vi "tap_stim_rec_async.vi"(0 "Convert Power to Voltage B":bool, 2 "voltages/power B":dbl[](array[numeric]), 3 "SSH password":string, 4 "Transfer and Run Date Folder After Experiment":bool, 5 "SSH user name":string, 6 "Tags":string, 7 "Frames":i32, 8 "Convert Power to Voltage A":bool, 9 "voltages/power A":dbl[](array[numeric]), 10 "parameters":string[](array[string]), 11 "parameters headers":string[](array[string])) -> ()   [LabVIEW 2019]
uses:
  <vilib>/Utility/file.llb/Write To Spreadsheet File (string).vi
  <vilib>/Utility/file.llb/Read From Spreadsheet File (string).vi
  <vilib>/vision/driver/IMAQdx.llb/IMAQdx Acquisition Mode.ctl
  <vilib>/vision/driver/NI_Vision_Acquisition_Software.lvlib
  <vilib>/userdefined/High Color/IMAQdx.ctl
  <vilib>/vision/driver/IMAQdx.llb/IMAQdx Buffer Number Mode.ctl
  <vilib>/Utility/file.llb/Write To Spreadsheet File (DBL).vi
panel:
  out "Saved Buffer Number":u32
  out "ProcessFrameRate":dbl
  out "# elements in queue":i32
  out "CameraFrameRate":dbl
  out "Camera Buffer Number":u32
  out "Image":T1(plugin-control)
  out "JPEG Quality":dbl
  out "Error":string
  out "Save Directory":path
  in  "stop":bool
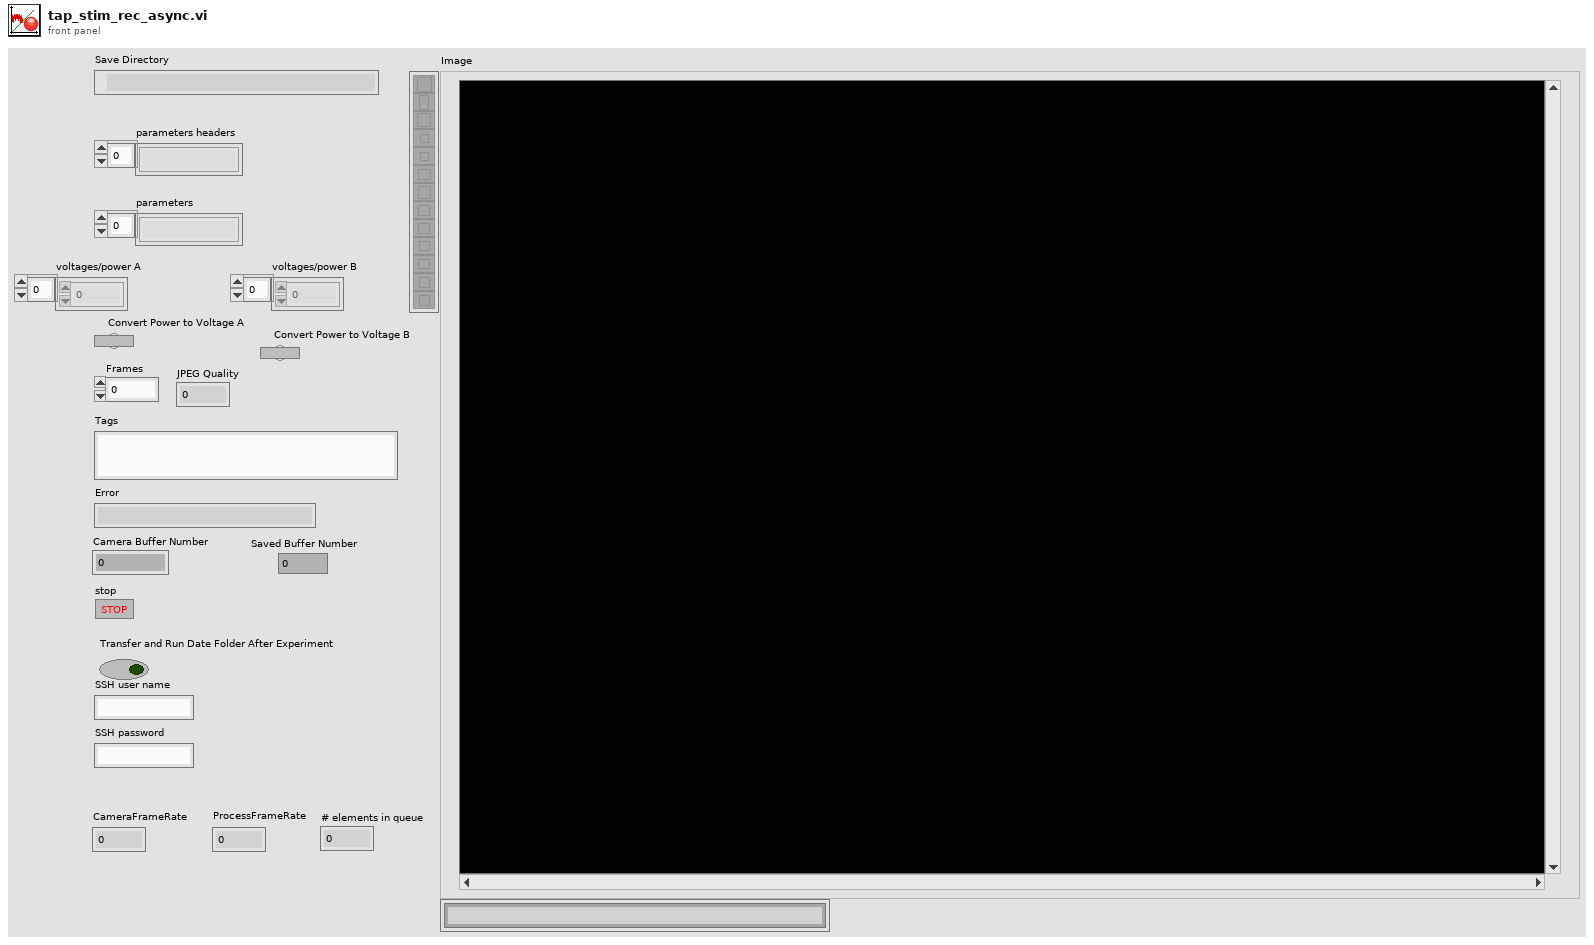
[diagram p1: front panel]
types:
  T1 = typedef "IMAQ Image.ctl" = refnum<image>
  T2 = typedef "IMAQdx.ctl" = refnum<k21>
  T3 = typedef "NI_Vision_Acquisition_Software.lvlib/IMAQdx Buffer Number Mode.ctl" = enum32{"Next", "Last", "Buffer Number", "Every", "Last New"}
  T4 = typedef "Image Type" = u32
  T5 = typedef "NI_Vision_Acquisition_Software.lvlib/IMAQdx Acquisition Mode.ctl" = enum32{"One Shot", "Continuous"}
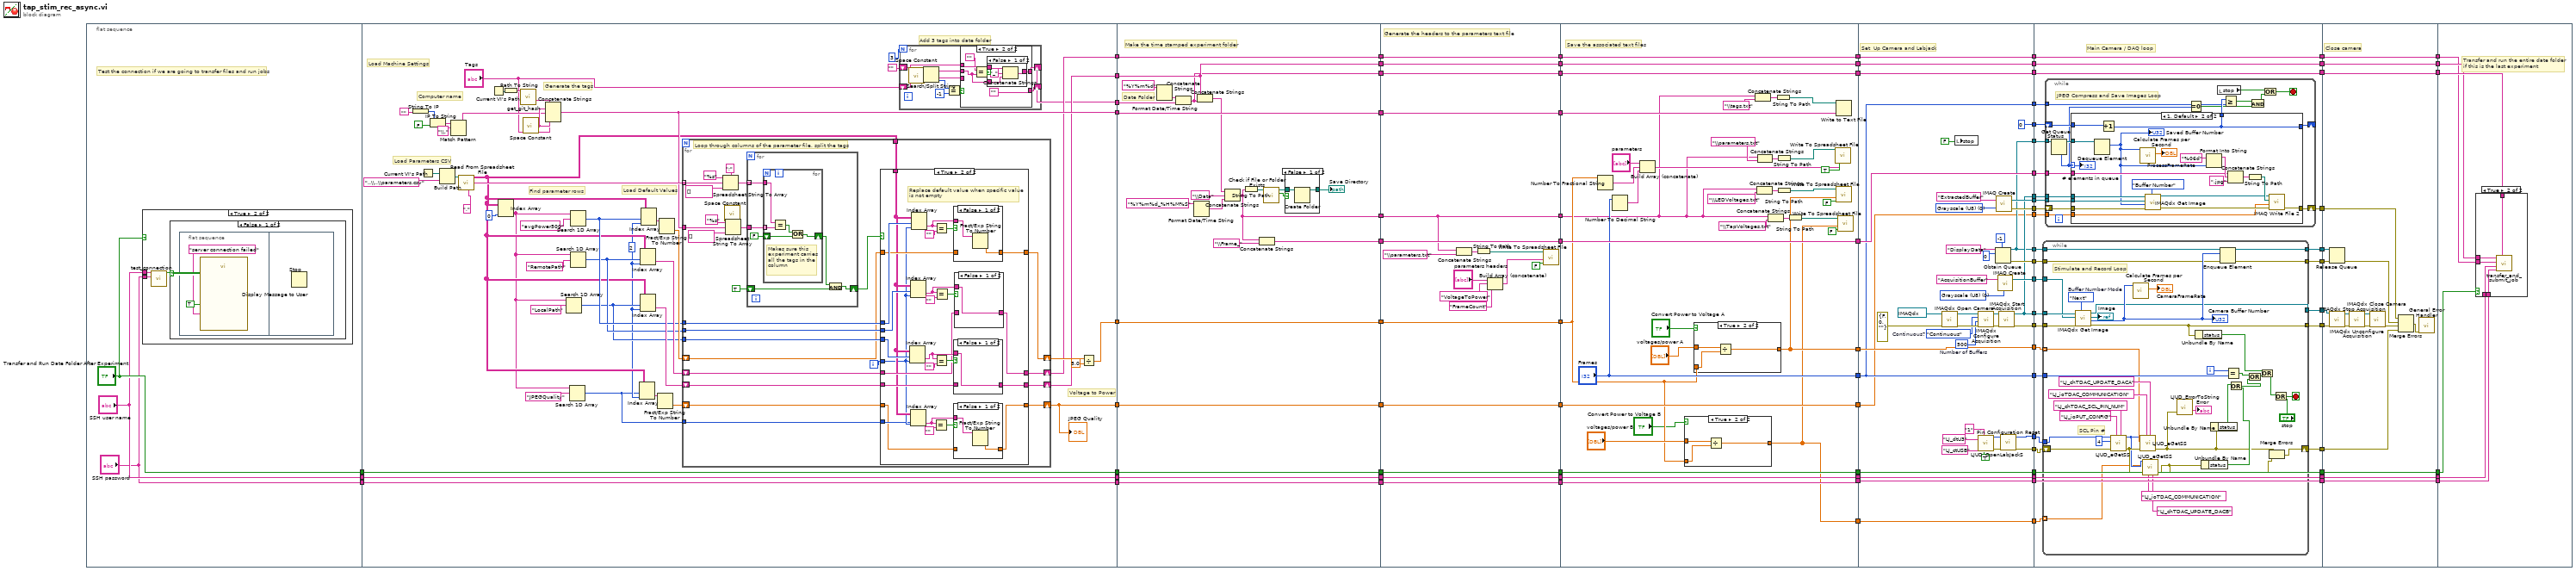
[diagram p0: block diagram]
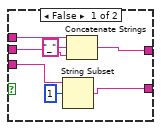
[diagram p4: hidden frame]
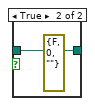
[diagram p11: hidden frame]
diagram:
  n1 = flat-sequence {
    tunnel: ["Transfer and Run Date Folder After Experiment"] -> w50
    tunnel: ["SSH user name"] -> w49
    tunnel: ["SSH password"] -> w48
    tunnel: [w134] -> w80
    tunnel: [w117] -> w79
    tunnel: [w108] -> w70
    tunnel: [w109] -> w69
    tunnel: w50 -> [w126]
    tunnel: w49 -> [w125]
    tunnel: w48 -> [w124]
    tunnel: [w126] -> w41
    tunnel: [w125] -> w34
    tunnel: [w124] -> w33
    tunnel: [w105] -> w26
    tunnel: [w96] -> w25
    tunnel: [w270] -> w64
    tunnel: [w269] -> w62
    tunnel: [w268] -> w60
    tunnel: [w267] -> w58
    tunnel: [w249] -> w56
    tunnel: [w251] -> w54
    tunnel: [w266] -> w52
    tunnel: w69 -> [w266]
    tunnel: w70 -> [w251]
    tunnel: w79 -> [w267]
    tunnel: w80 -> [w268]
    tunnel: [w258] -> w42
    tunnel: w41 -> [w258]
    tunnel: [w257] -> w35
    tunnel: w34 -> [w257]
    tunnel: w33 -> [w256]
    tunnel: [w256] -> w32
    tunnel: w26 -> [w252]
    tunnel: w25 -> [w248]
    tunnel: [w248] -> w22
    tunnel: w64 -> [w292]
    tunnel: [w292] -> w63
    tunnel: w62 -> [w278]
    tunnel: [w278] -> w61
    tunnel: w60 -> [w291]
    tunnel: [w291] -> w59
    tunnel: w58 -> [w290]
    tunnel: [w290] -> w57
    tunnel: w56 -> [w289]
    tunnel: [w289] -> w55
    tunnel: w54 -> [w288]
    tunnel: [w288] -> w53
    tunnel: w52 -> [w287]
    tunnel: [w287] -> w51
    tunnel: [w277] -> w43
    tunnel: w42 -> [w277]
    tunnel: [w276] -> w36
    tunnel: w35 -> [w276]
    tunnel: w32 -> [w275]
    tunnel: [w275] -> w31
    tunnel: [w274] -> w23
    tunnel: w22 -> [w274]
    tunnel: w63 -> [w327]
    tunnel: [w327] -> w85
    tunnel: [w298] -> w83
    tunnel: ["Frames"] -> w82
    tunnel: w61 -> [w294]
    tunnel: w59 -> [w301]
    tunnel: w57 -> [w305]
    tunnel: w55 -> [w316]
    tunnel: [w316] -> w75
    tunnel: [w315] -> w71
    tunnel: w53 -> [w315]
    tunnel: [w314] -> w65
    tunnel: w51 -> [w314]
    tunnel: [w308] -> w44
    tunnel: w43 -> [w308]
    tunnel: [w307] -> w37
    tunnel: w36 -> [w307]
    tunnel: w31 -> [w306]
    tunnel: [w306] -> w30
    tunnel: [w304] -> w24
    tunnel: w23 -> [w304]
    tunnel: [w293] -> w1
    tunnel: w85 -> [w344]
    tunnel: [w374] -> w87
    tunnel: [w373] -> w86
    tunnel: [w377] -> w84
    tunnel: w83 -> [w377]
    tunnel: w82 -> [w343]
    tunnel: [w343] -> w81
    tunnel: [w371] -> w76
    tunnel: w75 -> [w371]
    tunnel: [w370] -> w72
    tunnel: w71 -> [w370]
    tunnel: [w369] -> w66
    tunnel: w65 -> [w369]
    tunnel: [w368] -> w45
    tunnel: w44 -> [w368]
    tunnel: [w367] -> w38
    tunnel: w37 -> [w367]
    tunnel: w30 -> [w366]
    tunnel: [w366] -> w29
    tunnel: w24 -> [w341]
    tunnel: [w350] -> w21
    tunnel: [w345] -> w20
    tunnel: [w349] -> w19
    tunnel: [w348] -> w18
    tunnel: [w342] -> w17
    tunnel: [w347] -> w14
    tunnel: [w346] -> w13
    tunnel: [w345] -> w12
    tunnel: [w344] -> w11
    tunnel: [w343] -> w10
    tunnel: [w342] -> w9
    tunnel: [w341] -> w8
    tunnel: [0] -> w4
    tunnel: [w338] -> w2
    tunnel: w1 -> [w338]
    tunnel: w87 -> [w395]
    tunnel: w86 -> [w387]
    tunnel: w84 -> [w393]
    tunnel: w81 -> [w394]
    tunnel: [w410] -> w77
    tunnel: w76 -> [w410]
    tunnel: [w409] -> w73
    tunnel: w72 -> [w409]
    tunnel: [w408] -> w67
    tunnel: w66 -> [w408]
    tunnel: [w407] -> w46
    tunnel: w45 -> [w407]
    tunnel: [w406] -> w39
    tunnel: w38 -> [w406]
    tunnel: w29 -> [w405]
    tunnel: [w405] -> w28
    tunnel: w21 -> [w388]
    tunnel: w20 -> [w389]
    tunnel: w19 -> [w390]
    tunnel: w18 -> [w391]
    tunnel: w17 -> [w392]
    tunnel: [w383] -> w16
    tunnel: [w382] -> w15
    tunnel: w14 -> [w404]
    tunnel: w13 -> [w403]
    tunnel: w12 -> [w402]
    tunnel: w11 -> [w401]
    tunnel: w10 -> [w400]
    tunnel: w9 -> [w399]
    tunnel: w8 -> [w398]
    tunnel: [w381] -> w7
    tunnel: [w384] -> w6
    tunnel: [w397] -> w5
    tunnel: w4 -> [w396]
    tunnel: [w385] -> w3
    tunnel: w2 -> [w386]
    tunnel: [w509] -> w78
    tunnel: w77 -> [w509]
    tunnel: [w508] -> w74
    tunnel: w73 -> [w508]
    tunnel: [w507] -> w68
    tunnel: w67 -> [w507]
    tunnel: [w506] -> w47
    tunnel: w46 -> [w506]
    tunnel: [w505] -> w40
    tunnel: w39 -> [w505]
    tunnel: w28 -> [w504]
    tunnel: [w504] -> w27
    tunnel: w16 -> [w499]
    tunnel: w15 -> [w498]
    tunnel: w7 -> [w493]
    tunnel: w6 -> [w496]
    tunnel: w5 -> [w495]
    tunnel: w3 -> [w494]
    tunnel: w78 -> [w515]
    tunnel: w74 -> [w514]
    tunnel: w68 -> [w513]
    tunnel: w47 -> [w512]
    tunnel: w40 -> [w511]
    tunnel: w27 -> [w510]
    frame #0 {
      # "Test the connection if we are going to transfer files and run jobs"
      n2 = case shown="True" "Transfer and Run Date Folder After Experiment" {
        tunnel: "SSH password" -> [_ w93]
        tunnel: "SSH user name" -> [_ w91]
        frame False {
        }
        frame True {
          n3 = call "test_connection.vi"("Username"=w91, "Password"=w93) -> ("Connection Successful"=w92:bool)  [unwired: 7 in]
          n4 = case shown="False" w92 {
            frame False {
              n5 = flat-sequence {
                frame #0 {
                  n6 = call "Display Message to User"("Enable"=TRUE, "Message"="server connection failed") -> ()  [unwired: 8 in, 2 out]
                }
                frame #1 {
                  n7 = Stop() -> ()  [unwired: 1 in]
                }
              }
            }
            frame True {
            }
          }
        }
      }
    }
    frame #1 {
      w99 = 2
      # "Add 3 tags into date folder"
      # "Generate the tags"
      # "Find parameter rows"
      # "Load Default Values"
      # "Voltage to Power"
      # "Load Parameters CSV"
      # "Computer name"
      # "Load Machine Settings"
      n8 = String To IP(1:"") -> (0:w142:u32)
      n9 = Current VI's Path() -> (path=w137:path)
      n10 = IP To String(1:FALSE, 2:w142) -> (0:w139:string)
      n11 = Build Path(base path=w137, name or relative path="..\\..\\parameters.csv") -> (appended path=w128:path)
      n12 = Match Pattern(string=w139, regular expression="\\.") -> (before substring=w119:string)  [unwired: 1 in, 3 out]
      n13 = call-poly <vilib>:"Read From Spreadsheet File.vi"("delimiter (\\t)"=",", "file path (dialog if empty)"=w128) -> ("first row"=w118:string[], "all rows"=w101:string[][])  [unwired: 5 in, 3 out]
      n14 = Current VI's Path() -> (path=w121:path)
      n15 = Index Array(array=w101, index (col)=0) -> (element=w100:string[])  [unwired: 1 in]
      n16 = Path To String(path=w121) -> (string=w120:string)
      n17 = call "get_git_hash.vi"("VI folder"=w120) -> ("github hash"=w123:string)  [unwired: 10 in]
      n18 = call <vilib>:"Space Constant.vi"() -> ("String"=w122:string)
      n19 = Concatenate Strings(w123, w122, w119, w122, "Tags") -> (w117:string)
      n20 = Search 1D Array(1D array=w100, element="LocalPath") -> (index of element=w111:i32)  [unwired: 1 in]
      n21 = Search 1D Array(1D array=w100, element="JPEGQuality") -> (index of element=w97:i32)  [unwired: 1 in]
      n22 = Search 1D Array(1D array=w100, element="RemotePath") -> (index of element=w112:i32)  [unwired: 1 in]
      n23 = Search 1D Array(1D array=w100, element="avgPower500") -> (index of element=w113:i32)  [unwired: 1 in]
      n24 = Index Array(array=w101, index (row)=w97, index (col)=w99) -> (element=w102:string)
      n25 = Index Array(array=w101, index (row)=w112, index (col)=w99) -> (element=w115:string)
      n26 = Index Array(array=w101, index (row)=w111, index (col)=w99) -> (element=w114:string)
      n27 = Index Array(array=w101, index (row)=w113, index (col)=w99) -> (element=w130:string)
      n28 = Fract/Exp String To Number(string=w102) -> (number=w98:dbl)  [unwired: 3 in, 1 out]
      n29 = Fract/Exp String To Number(string=w130) -> (number=w116:dbl)  [unwired: 3 in, 1 out]
      n30 = for {
        tunnel: w118 -> [w196] mode=indexing
        tunnel: w117 -> [w188]
        tunnel: w113 -> [w183]
        tunnel: w112 -> [w182]
        tunnel: w111 -> [w181]
        tunnel: w101 -> [w186]
        shift-right: [w178] -> w110
        shift-left: w116 -> [w179]
        shift-right: [w175] -> w109
        shift-left: w115 -> [w176]
        shift-right: [w174] -> w108
        shift-left: w114 -> [w177]
        shift-right: [w171] -> w96
        shift-left: w98 -> [w173]
        tunnel: w97 -> [w172]
        i -> [w180]
        # "Loop through columns of the parameter file, split the tags"
        n31 = Spreadsheet String To Array(delimiter (Tab)=";", format string="%s", spreadsheet string=w196, array type (2D Dbl)=string[] []) -> (array=w192:string[])
        n32 = call <vilib>:"Space Constant.vi"() -> ("String"=w190:string)
        n33 = Spreadsheet String To Array(delimiter (Tab)=w190, format string="%s", spreadsheet string=w188, array type (2D Dbl)=string[] []) -> (array=w187:string[])
        n34 = for {
          tunnel: w192 -> [w242] mode=indexing
          tunnel: w187 -> [w241]
          shift-right: [w239] -> w184
          shift-left: TRUE -> [w237]
          n35 = for {
            tunnel: w242 -> [w247]
            tunnel: w241 -> [w246] mode=indexing
            shift-right: [w243] -> w238
            shift-left: FALSE -> [w244]
            # "Makes sure this\nexperiment carries\nall the tags in the\ncolumn"
            n36 = Equal?(x=w247, y=w246) -> (x = y?=w245:bool)
            n37 = Or(x=w245, y=w244) -> (x .or. y?=w243:bool)
          }
          n38 = And(x=w238, y=w237) -> (x .and. y?=w239:bool)
        }
        n39 = case shown="True" w184 {
          tunnel: w179 -> [w200 w221]
          tunnel: [w200 w220] -> w178
          tunnel: w183 -> [_ w226]
          tunnel: w182 -> [_ w225]
          tunnel: w181 -> [_ w224]
          tunnel: w180 -> [_ w203]
          tunnel: w186 -> [_ w204]
          tunnel: [w199 w210] -> w175
          tunnel: [w198 w212] -> w174
          tunnel: w177 -> [w198 w211]
          tunnel: w176 -> [w199 w209]
          tunnel: w173 -> [w197 w201]
          tunnel: w172 -> [_ w202]
          tunnel: [w197 w205] -> w171
          frame False {
          }
          frame True {
            # "Replace default value when specific value\nis not empty"
            n40 = Index Array(array=w204, index (row)=w224, index (col)=w203) -> (element=w213:string)
            n41 = Index Array(array=w204, index (row)=w225, index (col)=w203) -> (element=w216:string)
            n42 = Index Array(array=w204, index (row)=w202, index (col)=w203) -> (element=w206:string)
            n43 = Index Array(array=w204, index (row)=w226, index (col)=w203) -> (element=w219:string)
            n44 = Equal?(x=w206, y="") -> (x = y?=w207:bool)
            n45 = Equal?(x=w219, y="") -> (x = y?=w222:bool)
            n46 = Equal?(x=w213, y="") -> (x = y?=w214:bool)
            n47 = Equal?(x=w216, y="") -> (x = y?=w217:bool)
            n48 = case shown="False" w207 {
              tunnel: w201 -> [_ w229]
              tunnel: [w228 w229] -> w205
              tunnel: w206 -> [w227 _]
              frame False {
                n49 = Fract/Exp String To Number(string=w227) -> (number=w228:dbl)  [unwired: 3 in, 1 out]
              }
              frame True {
              }
            }
            n50 = case shown="False" w222 {
              tunnel: w221 -> [_ w236]
              tunnel: [w235 w236] -> w220
              tunnel: w219 -> [w234 _]
              frame False {
                n51 = Fract/Exp String To Number(string=w234) -> (number=w235:dbl)  [unwired: 3 in, 1 out]
              }
              frame True {
              }
            }
            n52 = case shown="False" w214 {
              tunnel: w213 -> [w230 _]
              tunnel: [w230 w231] -> w212
              tunnel: w211 -> [_ w231]
              frame False {
              }
              frame True {
              }
            }
            n53 = case shown="False" w217 {
              tunnel: w216 -> [w232 _]
              tunnel: [w232 w233] -> w210
              tunnel: w209 -> [_ w233]
              frame False {
              }
              frame True {
              }
            }
          }
        }
      }
      "JPEG Quality" <- w96
      n54 = for {
        N: 3 -> [_]
        shift-right: [w143] -> _
        shift-left: "Tags" -> [w152]
        shift-right: [w145] -> w105
        shift-left: "" -> [w150]
        n55 = call <vilib>:"Space Constant.vi"() -> ("String"=w151:string)
        n56 = Search/Split String(string=w152, search string/char (-)=w151) -> (substring before match=w149:string, match + rest of string=w148:string, offset of match=w147:i32)  [unwired: 1 in]
        n57 = Equal?(x=w147, y=-1) -> (x = y?=w144:bool)
        n58 = case shown="True" w144 {
          tunnel: w150 -> [w153 w163]
          tunnel: w149 -> [w154 w160]
          tunnel: w148 -> [w155 _]
          tunnel: [w157 ""] -> w143
          tunnel: [w156 w162] -> w145
          frame False {
            n59 = String Subset(string=w155, offset (0)=1) -> (substring=w157:string)  [unwired: 1 in]
            n60 = Concatenate Strings(w153, "_", w154) -> (w156:string)
          }
          frame True {
            n61 = Equal?(x="", y=w160) -> (x = y?=w164:bool)
            n62 = case shown="False" w164 {
              tunnel: w163 -> [w167 w170]
              tunnel: [w168 w170] -> w162
              tunnel: w160 -> [w166 _]
              frame False {
                n63 = Concatenate Strings(w167, "_", w166) -> (w168:string)
              }
              frame True {
              }
            }
          }
        }
      }
      n64 = Divide(x=w110, y=5.0) -> (x/y=w134:dbl)
    }
    frame #2 {
      # "Make the time stamped experiment folder"
      # "Date Folder"
      n65 = Format Date/Time String(time format string (%c)="%Y%m%d") -> (date/time string=w253:string)  [unwired: 2 in]
      n66 = Concatenate Strings(w253, w252) -> (w249:string)
      n67 = Format Date/Time String(time format string (%c)="%Y%m%d_%H%M%S") -> (date/time string=w255:string)  [unwired: 2 in]
      n68 = Concatenate Strings(w251, w249) -> (w250:string)
      n69 = Concatenate Strings(w250, "\\Data", w255) -> (w269:string)
      n70 = String To Path(string=w269) -> (path=w261:path)
      n71 = Concatenate Strings(w269, "\\Frame_") -> (w270:string)
      n72 = call <vilib>:"Check if File or Folder Exists.vi"("path"=w261) -> ("file or folder exists?"=w264:bool, "dup path"=w263:path)  [unwired: 8 in, 1 out]
      n73 = case shown="False" w264 {
        tunnel: [w271 w273] -> w260
        tunnel: w263 -> [w272 w273]
        frame False {
          n74 = Create Folder(path (use dialog)=w272) -> (created path=w271:path)  [unwired: 2 in, 2 out]
        }
        frame True {
          (unwired) errorcluster {"status"=FALSE, "code"=0, "source"=""} ("error out")
        }
      }
      "Save Directory" <- w260
    }
    frame #3 {
      # "Generate the headers to the parameters text file"
      n75 = Concatenate Strings(w278, "\\parameters.txt") -> (w286:string)
      n76 = String To Path(string=w286) -> (path=w285:path)
      n77 = Build Array (concatenate)("parameters headers", "VoltageToPower", "FrameCount") -> (w282:string[])
      n78 = call-poly <vilib>:"Write To Spreadsheet File.vi"("append to file? (new file:F)"=FALSE, "1D data"=w282, "file path (dialog if empty)"=w285) -> ()  [unwired: 5 in, 1 out]
    }
    frame #4 {
      # "Save the associated text files"
      n79 = Number To Fractional String(number=w301) -> (F-format string=w310:string)  [unwired: 3 in]
      n80 = Number To Decimal String(number="Frames") -> (decimal integer string=w311:string)  [unwired: 1 in]
      n81 = Build Array (concatenate)("parameters", w310, w311) -> (w320:string[])
      n82 = case shown="True" "Convert Power to Voltage B" {
        tunnel: "voltages/power B" -> [w330 w333]
        tunnel: [w330 w331] -> w293
        tunnel: w301 -> [_ w332]
        frame False {
        }
        frame True {
          n83 = Divide(x=w333, y=w332) -> (x/y=w331:dbl[])
        }
      }
      n84 = case shown="True" "Convert Power to Voltage A" {
        tunnel: "voltages/power A" -> [w334 w337]
        tunnel: [w334 w335] -> w298
        tunnel: w301 -> [_ w336]
        frame False {
        }
        frame True {
          n85 = Divide(x=w337, y=w336) -> (x/y=w335:dbl[])
        }
      }
      n86 = Concatenate Strings(w294, "\\tags.txt") -> (w318:string)
      n87 = Concatenate Strings(w294, "\\LEDVoltages.txt") -> (w329:string)
      n88 = Concatenate Strings(w294, "\\parameters.txt") -> (w324:string)
      n89 = Concatenate Strings(w294, "\\TapVoltages.txt") -> (w297:string)
      n90 = String To Path(string=w318) -> (path=w317:path)
      n91 = String To Path(string=w329) -> (path=w328:path)
      n92 = String To Path(string=w324) -> (path=w323:path)
      n93 = String To Path(string=w297) -> (path=w295:path)
      n94 = call-poly <vilib>:"Write To Spreadsheet File.vi"("append to file? (new file:F)"=TRUE, "1D data"=w320, "file path (dialog if empty)"=w323) -> ()  [unwired: 5 in, 1 out]
      n95 = call-poly <vilib>:"Write To Spreadsheet File.vi"("append to file? (new file:F)"=FALSE, "1D data"=w298, "file path (dialog if empty)"=w328) -> ()  [unwired: 5 in, 1 out]
      n96 = Write to Text File(file (use dialog)=w317, text=w305) -> ()  [unwired: 2 in, 3 out]
      n97 = call-poly <vilib>:"Write To Spreadsheet File.vi"("append to file? (new file:F)"=FALSE, "1D data"=w293, "file path (dialog if empty)"=w295) -> ()  [unwired: 5 in, 1 out]
    }
    frame #5 {
      w353 = T4 0 items=["Grayscale (U8)", "Grayscale (I16)", "Grayscale (SGL)", "Complex (CSG)", "RGB (U32)", "HSL (U32)", "RGB (U64)"] ("Image Type")
      w362 = T4 0 items=["Grayscale (U8)", "Grayscale (I16)", "Grayscale (SGL)", "Complex (CSG)", "RGB (U32)", "HSL (U32)", "RGB (U64)"] ("Image Type")
      w363 = u32 500  # Number of Buffers
      w359 = IMAQdx_Acquisition_Mode."Continuous"  # Continuous?
      # "Set  Up Camera and Labjack"
      n98 = call <vilib>:"IMAQdx Open Camera.vi"("error in"=errorcluster {"status"=FALSE, "code"=0, "source"=""}, "Session In"=T2 "cam0") -> ("error out"=w364:errorcluster, "Session Out"=w365:T2)  [unwired: 8 in]
      n99 = local write "stop"(FALSE) -> ()
      n100 = call "LJUD_OpenLabJackS.vi"("FirstFound"=TRUE, "Address"="1" ("DeviceType"), "ConnectionType"="LJ_ctUSB", "DeviceType"="LJ_dtU3") -> ("error out"=w372:errorcluster, "Handle"=w375:i32)  [unwired: 5 in, 1 out]
      n101 = call <vilib>:"IMAQdx Configure Acquisition.vi"("error in"=w364, "Number of Buffers"=w363, "Continuous?"=w359, "Session In"=w365) -> ("error out"=w360:errorcluster, "Session Out"=w358:T2)  [unwired: 6 in]
      n102 = Obtain Queue(max queue size (-1, unlimited)=-1, name (unnamed)="DisplayData", element data type=u32 0) -> (queue out=w342:refnum<queue>, error out=w348:errorcluster)  [unwired: 2 in, 1 out]
      n103 = call "IMAQ Create"("Image Name"="ExtractedBuffer", "Image Type"=w353) -> ("New Image"=w346:T1, "error out"=w347:errorcluster)  [unwired: 3 in]
      n104 = call "IMAQ Create"("Image Name"="AcquisitionBuffer", "Image Type"=w362) -> ("New Image"=w349:T1)  [unwired: 3 in, 1 out]
      n105 = call <vilib>:"IMAQdx Start Acquisition.vi"("error in"=w360, "Session In"=w358) -> ("error out"=w350:errorcluster, "Session Out"=w345:T2)  [unwired: 8 in]
      n106 = call "Pin Configuration Reset.vi"("error in"=w372, "Handle In"=w375) -> ("error out"=w373:errorcluster, "Handle Out"=w374:i32)  [unwired: 8 in]
    }
    frame #6 {
      # "Main Camera / DAQ loop"
      n107 = while {
        shift-right: [w411] -> w381
        shift-left: w387 -> [w440]
        tunnel: w393 -> [w439] mode=indexing
        tunnel: w394 -> [w446]
        tunnel: w388 -> [w434]
        tunnel: w389 -> [w433]
        tunnel: w390 -> [w432]
        tunnel: w391 -> [w431]
        tunnel: w392 -> [w430]
        tunnel: [w426] -> w385
        tunnel: [w425] -> w384
        tunnel: [w424] -> w383
        tunnel: [w423] -> w382
        tunnel: w395 -> [w419]
        tunnel: w386 -> [w417] mode=indexing
        i -> [w447]
        stop <- w451 stop-if-true
        w438 = IMAQdx_Buffer_Number_Mode."Next"  # Buffer Number Mode
        # "Stimulate and Record Loop"
        # "SCL Pin #"
        n108 = call <vilib>:"IMAQdx Get Image.vi"("Buffer Number Mode (Next)"=w438, "error in"=w434, "Image In"=w432, "Session In"=w433) -> ("error out"=w423:errorcluster, "Buffer Number Out"=w435:u32, "Image Out"=→"Image":T1, "Session Out"=w424:T2)  [unwired: 4 in]
        "Camera Buffer Number" <- w435
        n109 = call "LJUD_eGetSS.vi"("Channel"="LJ_chTDAC_SCL_PIN_NUM", "IOType"="LJ_ioPUT_CONFIG", "error in"=w440, "Value Write"=4, "Handle In"=w419) -> ("error out"=w422:errorcluster, "Handle Out"=w418:i32)  [unwired: 4 in, 1 out]
        n110 = call <vilib>:"Calculate Frames per Second.vi"("Buffer Number"=w435) -> ("Processed Frames/s"=→"CameraFrameRate":dbl)  [unwired: 8 in, 2 out]
        n111 = call "LJUD_eGetSS.vi"("Channel"="LJ_chTDAC_UPDATE_DACA", "IOType"="LJ_ioTDAC_COMMUNICATION", "error in"=w422, "Value Write"=w439, "Handle In"=w418) -> ("error out"=w413:errorcluster)  [unwired: 4 in, 2 out]
        n112 = call "LJUD_eGetSS.vi"("Channel"="LJ_chTDAC_UPDATE_DACB", "IOType"="LJ_ioTDAC_COMMUNICATION", "error in"=w422, "Value Write"=w417, "Handle In"=w418) -> ("error out"=w412:errorcluster)  [unwired: 4 in, 2 out]
        n113 = call "LJUD_ErrorToString.vi"("error in"=w413) -> ("String"=→"Error":string)  [unwired: 10 in]
        n114 = Unbundle By Name(w423) -> ("status"=w429:bool)
        n115 = Unbundle By Name(w412) -> ("status"=w416:bool)
        n116 = Unbundle By Name(w413) -> ("status"=w415:bool)
        n117 = Enqueue Element(queue=w430, element=w435, error in (no error)=w431) -> (queue out=w426:refnum<queue>, error out=w425:errorcluster)  [unwired: 1 in, 1 out]
        n118 = Equal?(x=w447, y=w446) -> (x = y?=w448:bool)
        n119 = Or(x=w415, y=w416) -> (x .or. y?=w414:bool)
        n120 = Or(x=w448, y=w414) -> (x .or. y?=w428:bool)
        n121 = Or(x=w429, y=w428) -> (x .or. y?=w427:bool)
        n122 = Merge Errors(w413, w412) -> (w411:errorcluster)
        n123 = Or(x=w427, y="stop") -> (x .or. y?=w451:bool)
      }
      n124 = while {
        tunnel: w399 -> [w469]
        tunnel: w403 -> [w467]
        tunnel: w402 -> [w466]
        tunnel: w401 -> [w464]
        shift-right: [w463] -> w397
        shift-left: w404 -> [w465]
        tunnel: w400 -> [w456]
        tunnel: w398 -> [w461]
        shift-right: [w458] -> _
        shift-left: w396 -> [w459]
        stop <- w462 stop-if-true
        # "JPEG Compress and Save Images Loop"
        n125 = Get Queue Status(queue=w469) -> (queue out=w468:refnum<queue>, # elements in queue=w452:i32)  [unwired: 2 in, 6 out]
        n126 = case shown="1, Default" w452 {
          selector: w452 -> [_ w490]
          tunnel: w468 -> [_ w488]
          tunnel: w467 -> [_ w487]
          tunnel: w466 -> [_ w486]
          tunnel: w465 -> [w471 w485]
          tunnel: w464 -> [_ w479]
          tunnel: [w471 w475] -> w463
          tunnel: w461 -> [_ w474]
          tunnel: w459 -> [w470 w473]
          tunnel: [w470 w472] -> w458
          tunnel: [w470 w472] -> w457
          frame 0 {
          }
          frame 1, Default {
            n127 = Dequeue Element(queue=w488) -> (element=w476:u32)  [unwired: 2 in, 3 out]
            "Saved Buffer Number" <- w476
            n128 = Increment(x=w473) -> (x+1=w472:i32)
            n129 = call <vilib>:"Calculate Frames per Second.vi"("Buffer Number"=w476) -> ("Processed Frames/s"=→"ProcessFrameRate":dbl)  [unwired: 8 in, 2 out]
            n130 = call <vilib>:"IMAQdx Get Image.vi"("Buffer Number Mode (Next)"=IMAQdx_Buffer_Number_Mode."Buffer Number", "error in"=w485, "Buffer Number In"=w476, "Image In"=w487, "Session In"=w486) -> ("error out"=w477:errorcluster, "Image Out"=w478:T1)  [unwired: 3 in, 2 out]
            n131 = Format Into String(format string="%06d" ("string"), w476) -> (resulting string=w481:string)  [unwired: 2 in, 1 out]
            n132 = Concatenate Strings(w479, w481, ".jpg" ("string")) -> (w483:string)
            n133 = String To Path(string=w483) -> (path=w482:path)
            n134 = call-poly "IMAQ Write File 2"("error in (no error)"=w477, "Image Quality"=w474, "File Path"=w482, "Image"=w478) -> ("error out"=w475:errorcluster)  [unwired: 6 in, 1 out]
            "# elements in queue" <- w490
          }
        }
        n135 = Equal To 0?(x=w452) -> (x = 0?=w453:bool)
        n136 = local read "stop"() -> (w460:bool)
        n137 = Greater Or Equal?(x=w457, y=w456) -> (x >= y?=w455:bool)
        n138 = And(x=w455, y=w453) -> (x .and. y?=w454:bool)
        n139 = Or(x=w460, y=w454) -> (x .or. y?=w462:bool)
      }
    }
    frame #7 {
      # "Close camera"
      n140 = Release Queue(queue=w494) -> ()  [unwired: 2 in, 3 out]
      n141 = call <vilib>:"IMAQdx Stop Acquisition.vi"("error in"=w498, "Session In"=w499) -> ("error out"=w500:errorcluster, "Session Out"=w501:T2)  [unwired: 8 in]
      n142 = call <vilib>:"IMAQdx Unconfigure Acquisition.vi"("error in"=w500, "Session In"=w501) -> ("error out"=w503:errorcluster, "Session Out"=w502:T2)  [unwired: 8 in]
      n143 = call <vilib>:"IMAQdx Close Camera.vi"("error in"=w503, "Session In"=w502) -> ("error out"=w492:errorcluster)  [unwired: 9 in]
      n144 = Merge Errors(w495, w496, w492, w493) -> (w497:errorcluster)
      n145 = call <vilib>:"General Error Handler.vi"("error in (no error)"=w497) -> ()  [unwired: 10 in, 5 out]
    }
    frame #8 {
      # "Transfer and run the entire date folder\nif this is the last experiment"
      n146 = case shown="True" w512 {
        tunnel: w515 -> [_ w520]
        tunnel: w514 -> [_ w519]
        tunnel: w513 -> [_ w518]
        tunnel: w511 -> [_ w517]
        tunnel: w510 -> [_ w516]
        frame False {
        }
        frame True {
          n147 = call "transfer_and_submit_job.vi"("Date Folder"=w520, "Password"=w516, "Username"=w517, "Remote Data Directory"=w518, "Local Data Directory"=w519) -> ()  [unwired: 7 in]
        }
      }
    }
  }
